vi "Network.vi"() -> ()   [LabVIEW 2018]
uses:
  <extravilib>/ChannelInstances/Tag-c(bool,i32,str)/Write With Abort.vi
  <extravilib>/ChannelInstances/Tag-c(bool,i32,str)/Read With Abort.vi
  <extravilib>/ChannelInstances/Tag-c(bool,i32,str)/Instantiate.vi
  <extravilib>/ChannelInstances/Tag-c(bool,i32,str)/EndpointRead.vi
  <extravilib>/ChannelInstances/Tag-c(bool,i32,str)/Endpoint.vi
  <extravilib>/ChannelInstances/Tag-c(bool,i32,str).lvlib
panel:
  out "Temperature 1":dbl
  in  "Abort":bool
  in  "Launch":bool
  in  "Ready To Launch":bool
  in  "Send":bool
  out "Connected":bool
  in  "Command":string
  out "Fault Count":i32
  out "Fault Codes":string
  out "Report":string
  out "Distance":i32
  out "Current State":string
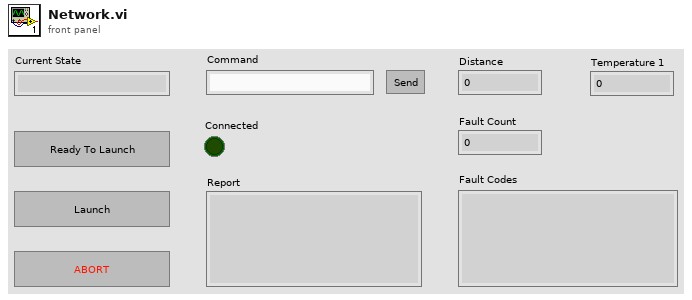
[diagram p1: front panel]
types:
  T1 = enum16{"Standard", "Buffered", "CRLF", "Immediate"}
  T2 = typedef "Tag-c(bool,i32,str).lvlib/))Channel.ctl" = refnum<queue>
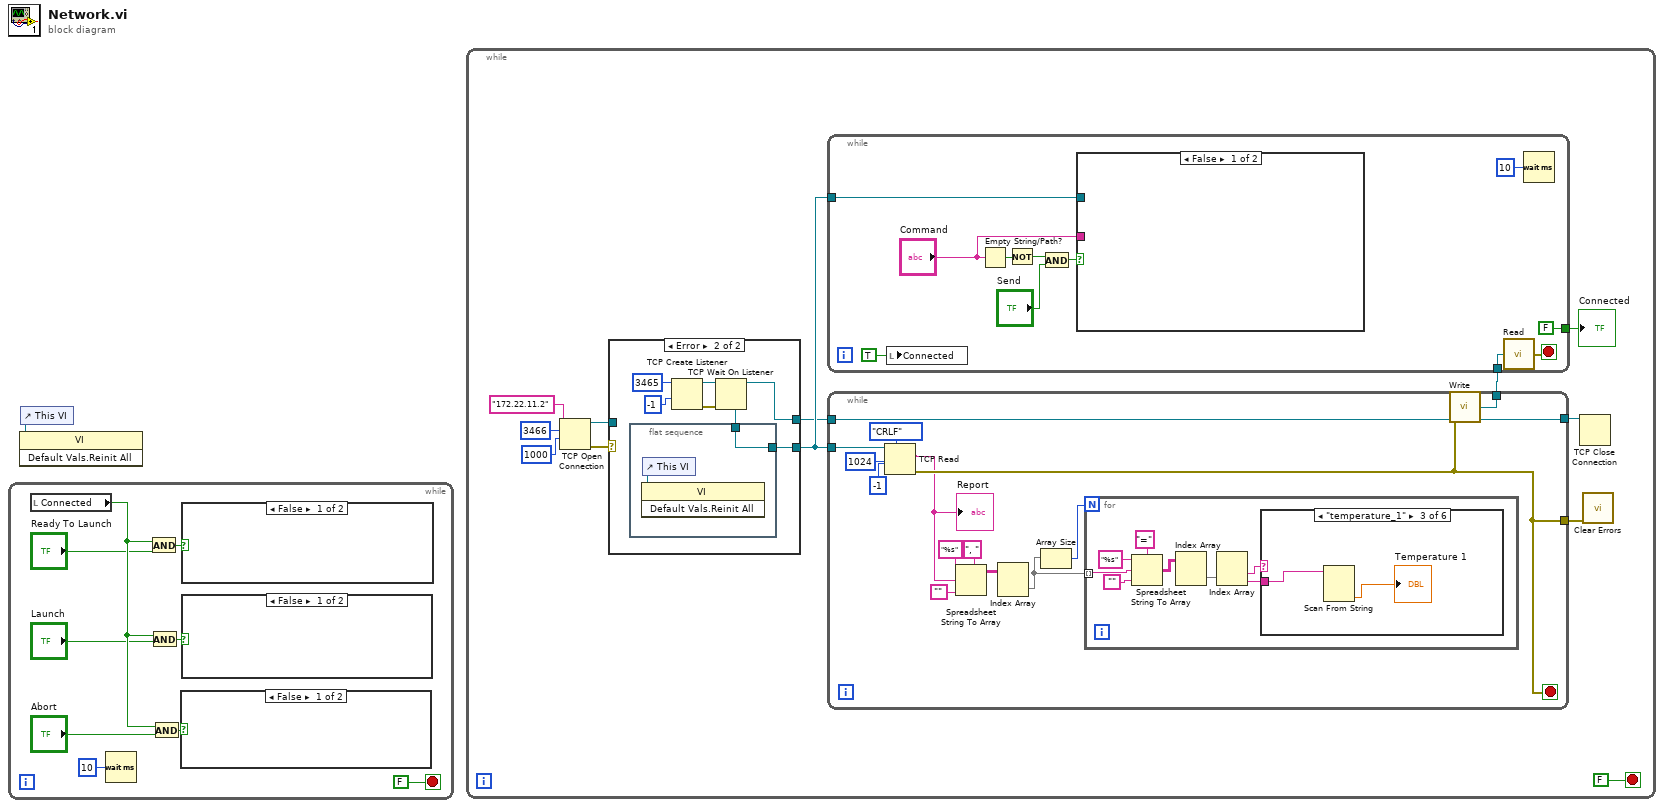
[diagram p0: block diagram]
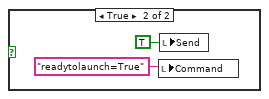
[diagram p2: hidden frame]
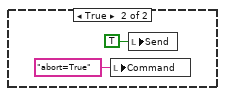
[diagram p3: hidden frame]
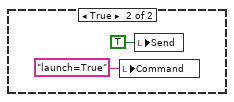
[diagram p4: hidden frame]
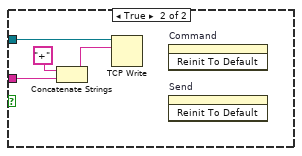
[diagram p6: hidden frame]
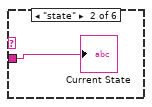
[diagram p8: hidden frame]
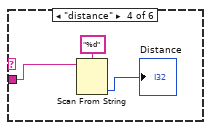
[diagram p9: hidden frame]
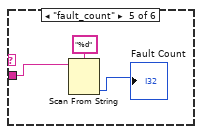
[diagram p10: hidden frame]
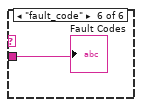
[diagram p11: hidden frame]
diagram:
  n1 = while {
    stop <- FALSE stop-if-true
    n2 = local read "Connected"() -> (w6:bool)
    n3 = Wait (ms)(milliseconds to wait=u32 10) -> ()  [unwired: 1 out]
    n4 = And(x=w6, y="Ready To Launch") -> (x .and. y?=w9:bool)
    n5 = And(x=w6, y="Launch") -> (x .and. y?=w8:bool)
    n6 = And(x=w6, y="Abort") -> (x .and. y?=w7:bool)
    n7 = case shown="False" w7 {
      frame False {
      }
      frame True {
        n8 = local write "Command"("abort=True") -> ()
        n9 = local write "Send"(TRUE ("Send")) -> ()
      }
    }
    n10 = case shown="False" w9 {
      frame False {
      }
      frame True {
        n11 = local write "Command"("readytolaunch=True") -> ()
        n12 = local write "Send"(TRUE ("Send")) -> ()
      }
    }
    n13 = case shown="False" w8 {
      frame False {
      }
      frame True {
        n14 = local write "Command"("launch=True") -> ()
        n15 = local write "Send"(TRUE ("Send")) -> ()
      }
    }
  }
  n16 = control-ref of="This VI"() -> (w1:refnum<vi>)
  n17 = invoke class="VI" method="Default Vals.Reinit All"(reference=w1) -> ()  [unwired: 2 in, 3 out]
  n18 = while {
    stop <- FALSE stop-if-true
    n19 = TCP Open Connection(address="172.22.11.2", remote port or service name=u16 3466, timeout ms (60000)=1000) -> (connection ID=w18:refnum<k5>, error out=w19:errorcluster)  [unwired: 2 in]
    n20 = case shown="Error" w19 {
      tunnel: [w29 w36] -> w25
      tunnel: [w29 w35] -> w23
      tunnel: w18 -> [w29 _]
      frame No Error {
      }
      frame Error {
        n21 = flat-sequence {
          tunnel: [w37] -> w36
          tunnel: w30 -> [w37]
          frame #0 {
            n22 = control-ref of="This VI"() -> (w38:refnum<vi>)
            n23 = invoke class="VI" method="Default Vals.Reinit All"(reference=w38) -> ()  [unwired: 2 in, 3 out]
          }
        }
        n24 = TCP Create Listener(9:-1 ("timeout ms (25000)"), 10:u16 3465 ("port")) -> (0:w33:errorcluster, 3:w34:refnum<k5>)  [unwired: 3 in, 1 out]
        n25 = TCP Wait On Listener(8:w33, 11:w34) -> (3:w35:refnum<k5>, 4:w30:refnum<k5>)  [unwired: 2 in, 3 out]
      }
    }
    n26 = while {
      tunnel: [w57] -> w24
      tunnel: [w58] -> w28
      tunnel: w25 -> [w55]
      tunnel: w23 -> [w54]
      tunnel: [w54] -> w22
      stop <- w57 stop-if-true
      n27 = TCP Read(connection ID=w55, bytes to read=1024, 7:T1."CRLF" ("mode (standard)"), 9:-1 ("timeout ms (25000)")) -> (data out=w56:string, error out=w57:errorcluster)  [unwired: 1 in, 1 out]
      "Report" <- w56
      n28 = Spreadsheet String To Array(delimiter (Tab)=", ", format string="%s", spreadsheet string=w56, array type (2D Dbl)="") -> (array=w64:string[][])
      n29 = Index Array(array=w64) -> (element=w62:string[])  [unwired: 2 in]
      n30 = Array Size(array=w62) -> (size(s)=w63:i32)
      n31 = for {
        N: w63 -> [_]
        tunnel: w62 -> [w70] mode=indexing
        n32 = Spreadsheet String To Array(delimiter (Tab)="=", format string="%s", spreadsheet string=w70, array type (2D Dbl)="") -> (array=w74:string[][])
        n33 = Index Array(array=w74) -> (element=w75:string[])  [unwired: 2 in]
        n34 = Index Array(array=w75) -> (element #1=w69:string, element #2=w68:string)  [unwired: 2 in]
        n35 = case shown="\"temperature_1\"" w69 {
          tunnel: w68 -> [_ w76 w78 w81 w84 w85]
          frame "False", Default {
          }
          frame "state" {
            "Current State" <- w76
          }
          frame "temperature_1" {
            n36 = Scan From String(input string=w78) -> (output 1=→"Temperature 1":dbl)  [unwired: 4 in, 3 out]
          }
          frame "distance" {
            n37 = Scan From String(format string="%d", input string=w81) -> (output 1=→"Distance":i32)  [unwired: 3 in, 3 out]
          }
          frame "fault_count" {
            n38 = Scan From String(format string="%d", input string=w84) -> (output 1=→"Fault Count":i32)  [unwired: 3 in, 3 out]
          }
          frame "fault_code" {
            "Fault Codes" <- w85
          }
        }
      }
      n39 = call <extravilib>:"Write.vi"("element"=w57) -> ("channel"=w58:T2)  [unwired: 1 out]
    }
    n40 = while {
      tunnel: w28 -> [w46]
      tunnel: [FALSE ("Boolean")] -> w26
      tunnel: w25 -> [w39]
      stop <- w47 stop-if-true
      n41 = local write "Connected"(TRUE ("Boolean")) -> ()
      n42 = Empty String/Path?(string/path="Command") -> (empty?=w48:bool)
      n43 = Not(x=w48) -> (.not. x?=w43:bool)
      n44 = And(x=w43, y="Send") -> (x .and. y?=w41:bool)
      n45 = case shown="False" w41 {
        tunnel: "Command" -> [_ w52]
        tunnel: w39 -> [_ w53]
        frame False {
        }
        frame True {
          n46 = Concatenate Strings("+", w52) -> (w50:string)
          n47 = TCP Write(connection ID=w53, data in=w50) -> ()  [unwired: 2 in, 3 out]
          n48 = invoke on="Command" class="Str" method="Reinit To Default"() -> ()  [unwired: 3 in, 3 out]
          n49 = invoke on="Send" class="Bool (strict)" method="Reinit To Default"() -> ()  [unwired: 3 in, 3 out]
        }
      }
      n50 = call <extravilib>:"Read.vi"("channel"=w46) -> ("element"=w47:errorcluster)  [unwired: 1 in, 1 out]
      n51 = Wait (ms)(milliseconds to wait=u32 10) -> ()  [unwired: 1 out]
    }
    "Connected" <- w26
    n52 = TCP Close Connection(connection ID=w22) -> ()  [unwired: 2 in, 2 out]
    n53 = call <vilib>:"Clear Errors.vi"("error in (no error)"=w24) -> ()  [unwired: 5 in, 2 out]
  }
